vi "annualMetData.vi"(1 "MET Data.csv":path) -> (0 "Annual Met Data":dbl[][](array[numeric]))   [LabVIEW 2018]
uses:
  <vilib>/Utility/file.llb/Read Delimited Spreadsheet (DBL).vi
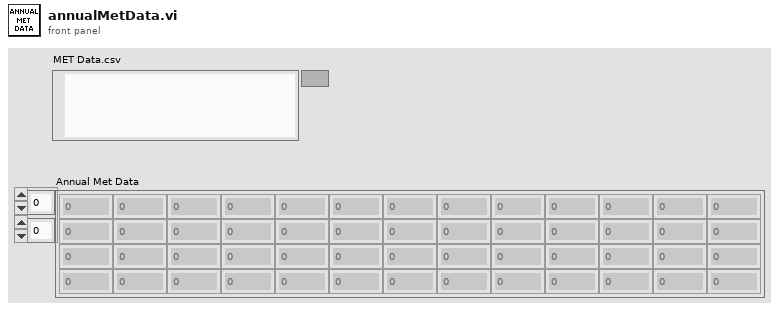
[diagram p1: front panel]
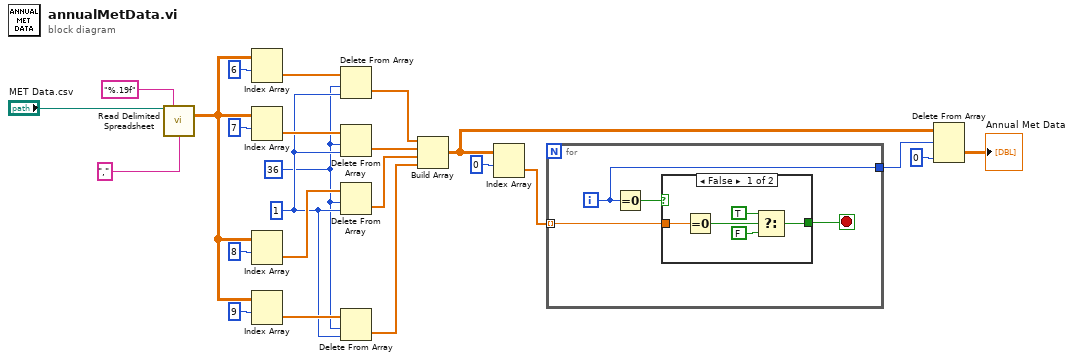
[diagram p0: block diagram]
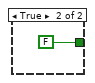
[diagram p2: hidden frame]
diagram:
  w11 = 36 ("length")
  w12 = 1 ("length")
  n1 = call-poly <vilib>:"Read Delimited Spreadsheet.vi"("file path (dialog if empty)"="MET Data.csv", "format (%.3f)"="%.19f", "delimiter (\\t)"="," ("delimiter (\\t)")) -> ("all rows"=w14:dbl[][])  [unwired: 7 in, 5 out]
  n2 = Index Array(array=w14, index (row)=6) -> (element=w13:dbl[])  [unwired: 1 in]
  n3 = Index Array(array=w14, index (row)=7) -> (element=w18:dbl[])  [unwired: 1 in]
  n4 = Index Array(array=w14, index (row)=8) -> (element=w17:dbl[])  [unwired: 1 in]
  n5 = Index Array(array=w14, index (row)=9) -> (element=w16:dbl[])  [unwired: 1 in]
  n6 = Delete From Array(array=w13, length=w11, index=w12) -> (deleted portion=w10:dbl[])  [unwired: 1 out]
  n7 = Delete From Array(array=w18, length=w11, index=w12) -> (deleted portion=w9:dbl[])  [unwired: 1 out]
  n8 = Delete From Array(array=w17, length=w11, index=w12) -> (deleted portion=w8:dbl[])  [unwired: 1 out]
  n9 = Delete From Array(array=w16, length=w11, index=w12) -> (deleted portion=w7:dbl[])  [unwired: 1 out]
  n10 = Build Array(w10, w9, w8, w7) -> (w4:dbl[][])
  n11 = Index Array(array=w4, index (row)=0 ("index")) -> (element=w5:dbl[])  [unwired: 1 in]
  n12 = for {
    tunnel: w5 -> [w25] mode=indexing
    tunnel: [w26] -> w2
    i -> [w26]
    stop <- w27 stop-if-true
    n13 = Equal To 0?(x=w26) -> (x = 0?=w28:bool)
    n14 = case shown="False" w28 {
      tunnel: w25 -> [w33 _]
      tunnel: [w29 FALSE] -> w27
      frame False {
        n15 = Equal To 0?(x=w33) -> (x = 0?=w32:bool)
        n16 = Select(t=TRUE, s=w32, f=FALSE) -> (s? t:f=w29:bool)
      }
      frame True {
      }
    }
  }
  n17 = Delete From Array(array=w4, length=w2, index (col)=0 ("index (row)")) -> (deleted portion=→"Annual Met Data":dbl[][])  [unwired: 1 in, 1 out]
